vi "MongoDB.CreateCollection.vi"(8 "error in (no error)":errorcluster, 10 "collectionName":string, 11 "MongoDB.Database in":refnum<class "MongoDB.Database.lvclass">) -> (0 "error out":errorcluster, 2 "MongoDB.Collection out":refnum<class "MongoDB.Collection.lvclass">, 3 "MongoDB.Database out":refnum<class "MongoDB.Database.lvclass">)   [LabVIEW 2014, in "MongoDB.Database.lvclass"]
uses:
  MongoDB.Database.lvclass
  MongoDB.Collection.lvclass
  MongoDB.Database.lvclass/MongoDB.Database.ctl
  C:/Users/Richard/Documents/GitHub/mongo-labview-driver/CSharp/bin/MongoDB.Driver.Legacy.dll
  CSharp/bin/MongoDB.Driver.Legacy.dll
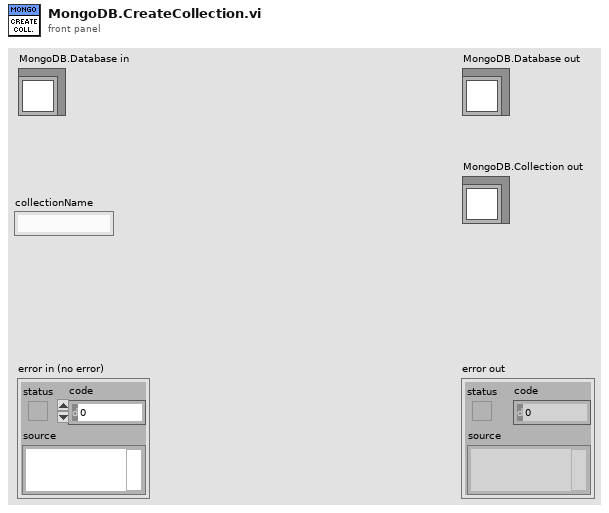
[diagram p1: front panel]
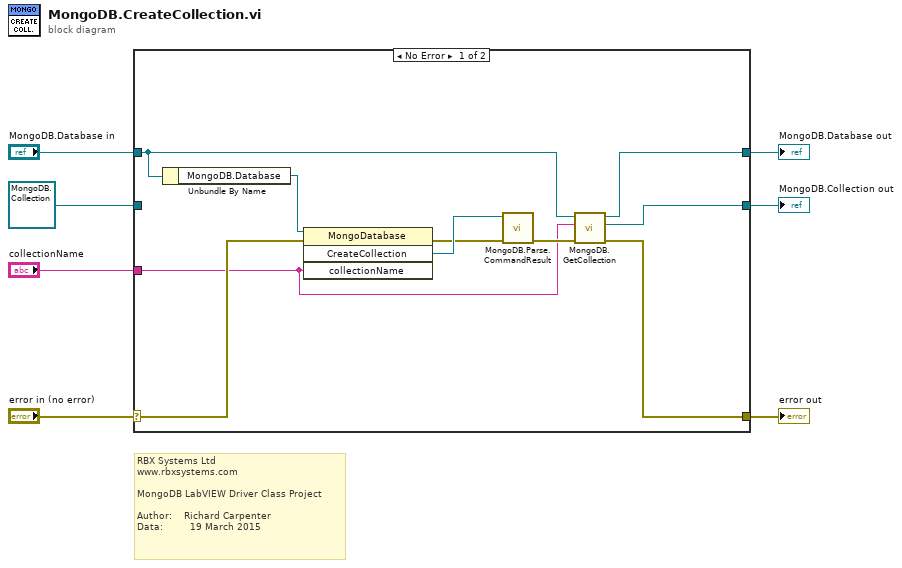
[diagram p0: block diagram]
diagram:
  # "RBX Systems Ltd\nwww.rbxsystems.com\n\nMongoDB LabVIEW Driver Class Project\n\nAuthor:    Richard Carpenter\nData:         19 March 2015"
  n1 = case shown="No Error" "error in (no error)" {
    selector: "error in (no error)" -> [w16 w20]
    tunnel: [w12 w20] -> w6
    tunnel: [w9 w19] -> w4
    tunnel: "MongoDB.Database in" -> [w10 w19]
    tunnel: [w11 w18] -> w3
    tunnel: refnum<class "MongoDB.Collection.lvclass"> refnum ("MongoDB.Collection in") -> [_ w18]
    tunnel: "collectionName" -> [w8 _]
    frame No Error {
      n2 = Unbundle By Name(w10) -> ("MongoDB.Database"=w17:refnum<k24>)
      n3 = invoke class="MongoDatabase" method="CreateCollection"(reference=w17, error in=w16, "collectionName"=w8) -> (error out=w14:errorcluster, "CreateCollection"=w15:refnum<k24>)  [unwired: 1 in, 2 out]
      n4 = call "MongoDB.Parse.CommandResult.vi"("error in (no error)"=w14, "MongoDB.Command.Result"=w15) -> ("error out"=w13:errorcluster)  [unwired: 9 in]
      n5 = call "MongoDB.GetCollection.vi"("error in (no error)"=w13, "collectionName"=w8, "MongoDB.Database in"=w10) -> ("error out"=w12:errorcluster, "MongoDB.Collection out"=w11:refnum<class "MongoDB.Collection.lvclass">, "MongoDB.Database out"=w9:refnum<class "MongoDB.Database.lvclass">)  [unwired: 6 in]
    }
    frame Error {
    }
  }
  "error out" <- w6
  "MongoDB.Database out" <- w4
  "MongoDB.Collection out" <- w3
